vi "Ref.vi"(7 "Event Actor in":refnum<class "Event Actor.lvclass">, 11 "String Indicator Ref in":refnum<class "String Indicator Ref.lvclass">) -> (5 "Event Actor out":refnum<class "Event Actor.lvclass">)   [LabVIEW 2021, in "String Indicator Ref.lvlib" / "String Indicator Ref.lvclass"]
uses:
  String Indicator Ref.lvclass
  Actor/Event Actor/Event Actor.lvclass
  String Indicator/String Indicator.lvclass
  String Indicator Ref.lvclass/String Indicator Ref.ctl
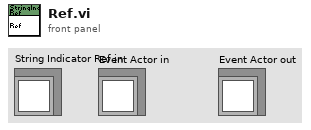
[diagram p1: front panel]
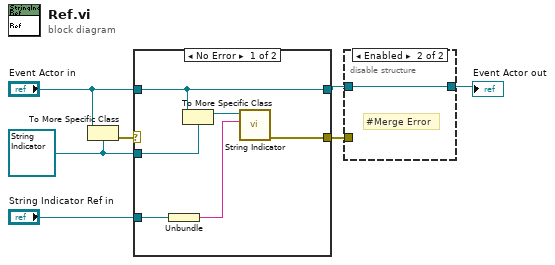
[diagram p0: block diagram]
diagram:
  w4 = refnum<class "String Indicator.lvclass"> refnum ("String Indicator Ref.lvlib:String Indicator.lvclass")
  n1 = To More Specific Class(target class=w4, reference="Event Actor in") -> (error out=w7:errorcluster)  [unwired: 1 in, 1 out]
  n2 = case shown="No Error" w7 {
    selector: w7 -> [_ w14]
    tunnel: [w10 w15] -> w2
    tunnel: "Event Actor in" -> [w10 w15]
    tunnel: w4 -> [w13 _]
    tunnel: "String Indicator Ref in" -> [w9 _]
    tunnel: [w11 w14] -> w1
    frame No Error {
      n3 = Unbundle(w9) -> (w8:string)
      n4 = To More Specific Class(target class=w13, reference=w10) -> (specific class reference=w12:refnum<class "String Indicator.lvclass">)  [unwired: 1 in, 1 out]
      n5 = call-dynamic "String Indicator.vi"("String Indicator"=w8, "String Indicator in"=w12) -> ("error out"=w11:errorcluster)  [unwired: 9 in]
    }
    frame Error {
    }
  }
  n6 = disable-structure shown="Enabled" {
    disable-tunnel: [w16 w17] -> w3
    disable-tunnel: w2 -> [w16 w17]
    disable-tunnel: w1 -> [_ _]
    frame Disabled {
    }
    frame Enabled {
      # "#Merge Error"
    }
  }
  "Event Actor out" <- w3
